vi "FdxCmdMonQueueSeekCvi.vi"(8 "error in":errorcluster, 9 "QueueSeekOut":T1 {"SeekOrigin" items=["FDX_SEEK_SET", "FDX_SEEK_END ", "FDX_SEEK_CUR", "FDX_SEEK_TRG"]}, 11 "InstrumentHandle_port":u32) -> (0 "error out":errorcluster, 1 "ByteOffset":i32, 3 "InstrumentHandle_port":u32)   [LabVIEW 2020, in "AIM664LV.lvlib"]
doc: "This function sets the read index to the data queue to read queue entries from a specified location.\nThis function is only applicable if the capture control is set to single (non-continuous)."
uses:
  AIM664LV.lvlib
  AFDX_LibraryAdmin/FdxGlobalDllPath.vi
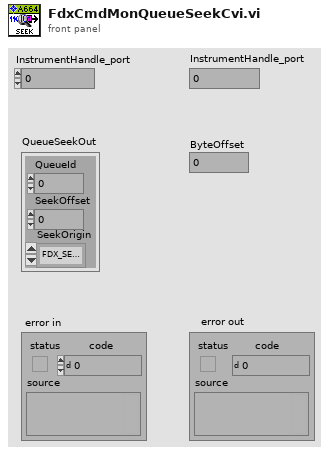
[diagram p1: front panel]
types:
  T1 = cluster{"QueueId":u32, "SeekOffset":i32, "SeekOrigin":u32}
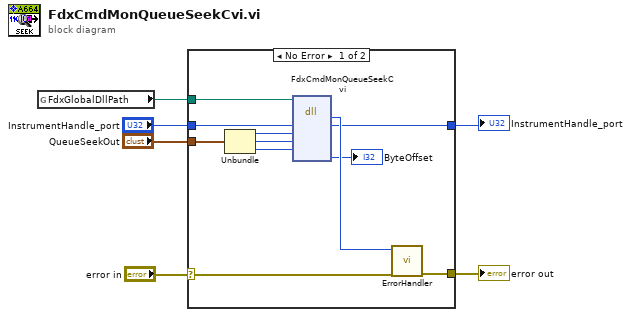
[diagram p0: block diagram]
diagram:
  n1 = global read "FdxGlobalDllPath.vi" "FdxGlobalDllPath"() -> (w4:path)
  n2 = case shown="No Error" "error in" {
    selector: "error in" -> [w16 w19]
    tunnel: [w17 w19] -> w6
    tunnel: w4 -> [w10 _]
    tunnel: "InstrumentHandle_port" -> [w9 w18]
    tunnel: [w8 w18] -> w2
    tunnel: "QueueSeekOut" -> [w7 _]
    frame No Error {
      n3 = Unbundle(w7) -> ("QueueId"=w13:u32, "SeekOffset"=w12:i32, "SeekOrigin"=w11:u32)
      n4 = dll-call lib="aim_fdx.19.dll" fn="FdxCmdMonQueueSeekCvi"(path in=w10, "InstrumentHandle"=w9, "QueueId"=w13, "SeekOffset"=w12, "SeekOrigin"=w11) -> ("status"=w15:i32, "InstrumentHandle"=w8:u32, "ByteOffset"=→"ByteOffset":i32)  [unwired: 5 in, 3 out]
      n5 = call "ErrorHandler.vi"("error in"=w16, "AIM Error"=w15) -> ("error out"=w17:errorcluster)  [unwired: 9 in]
    }
    frame Error {
    }
  }
  "error out" <- w6
  "InstrumentHandle_port" <- w2
